vi "Properties_Update RW From Value.vi"(11 "Properties for Tree In":T1(array[cluster])=[{"Label"="a", "Tag"="a", "Property Type"=enum."Base", "Indent"=0, "Can Read?"=TRUE, "Can Write?"=TRUE, "Is Read?"=FALSE, "Is Write?"=TRUE, "Inactive Parent?"=FALSE, "Unwired?"=FALSE}, {"Label"="b", "Tag"="b", "Property Type"=enum."Scripting", "Indent"=0, "Can Read?"=TRUE, "Can Write?"=FALSE, "Is Read?"=FALSE, "Is Write?"=FALSE, "Inactive Parent?"=FALSE, "Unwired?"=FALSE}, {"Label"="c", "Tag"="c", "Property Type"=enum."Base", "Indent"=0, "Can Read?"=TRUE, "Can Write?"=TRUE, "Is Read?"=FALSE, "Is Write?"=FALSE, "Inactive Parent?"=FALSE, "Unwired?"=FALSE}, {"Label"="d", "Tag"="d", "Property Type"=enum."Private", "Indent"=0, "Can Read?"=TRUE, "Can Write?"=FALSE, "Is Read?"=FALSE, "Is Write?"=FALSE, "Inactive Parent?"=FALSE, "Unwired?"=FALSE}, {"Label"="E", "Tag"="E", "Property Type"=enum."Base", "Indent"=0, "Can Read?"=TRUE, "Can Write?"=TRUE, "Is Read?"=FALSE, "Is Write?"=TRUE, "Inactive Parent?"=FALSE, "Unwired?"=FALSE}, {"Label"="f", "Tag"="f", "Property Type"=enum."Base", "Indent"=0, "Can Read?"=TRUE, "Can Write?"=FALSE, "Is Read?"=FALSE, "Is Write?"=FALSE, "Inactive Parent?"=FALSE, "Unwired?"=FALSE}]) -> (3 "Properties for Tree Out":T1(array[cluster])=[{"Label"="a", "Tag"="a", "Property Type"=enum."Base", "Indent"=0, "Can Read?"=TRUE, "Can Write?"=TRUE, "Is Read?"=FALSE, "Is Write?"=TRUE, "Inactive Parent?"=FALSE, "Unwired?"=FALSE}, {"Label"="b", "Tag"="b", "Property Type"=enum."Scripting", "Indent"=0, "Can Read?"=TRUE, "Can Write?"=FALSE, "Is Read?"=FALSE, "Is Write?"=FALSE, "Inactive Parent?"=FALSE, "Unwired?"=FALSE}, {"Label"="c", "Tag"="c", "Property Type"=enum."Base", "Indent"=0, "Can Read?"=TRUE, "Can Write?"=TRUE, "Is Read?"=FALSE, "Is Write?"=FALSE, "Inactive Parent?"=FALSE, "Unwired?"=FALSE}, {"Label"="d", "Tag"="d", "Property Type"=enum."Private", "Indent"=0, "Can Read?"=TRUE, "Can Write?"=FALSE, "Is Read?"=FALSE, "Is Write?"=FALSE, "Inactive Parent?"=FALSE, "Unwired?"=FALSE}, {"Label"="E", "Tag"="E", "Property Type"=enum."Base", "Indent"=0, "Can Read?"=TRUE, "Can Write?"=TRUE, "Is Read?"=FALSE, "Is Write?"=TRUE, "Inactive Parent?"=FALSE, "Unwired?"=FALSE}, {"Label"="f", "Tag"="f", "Property Type"=enum."Base", "Indent"=0, "Can Read?"=TRUE, "Can Write?"=FALSE, "Is Read?"=FALSE, "Is Write?"=FALSE, "Inactive Parent?"=FALSE, "Unwired?"=FALSE}])   [LabVIEW 2023]
doc: "Update properties array with current R/W status based on selection values.\n\nIf trees aren't already populated, the properties array is passed thorugh without change."
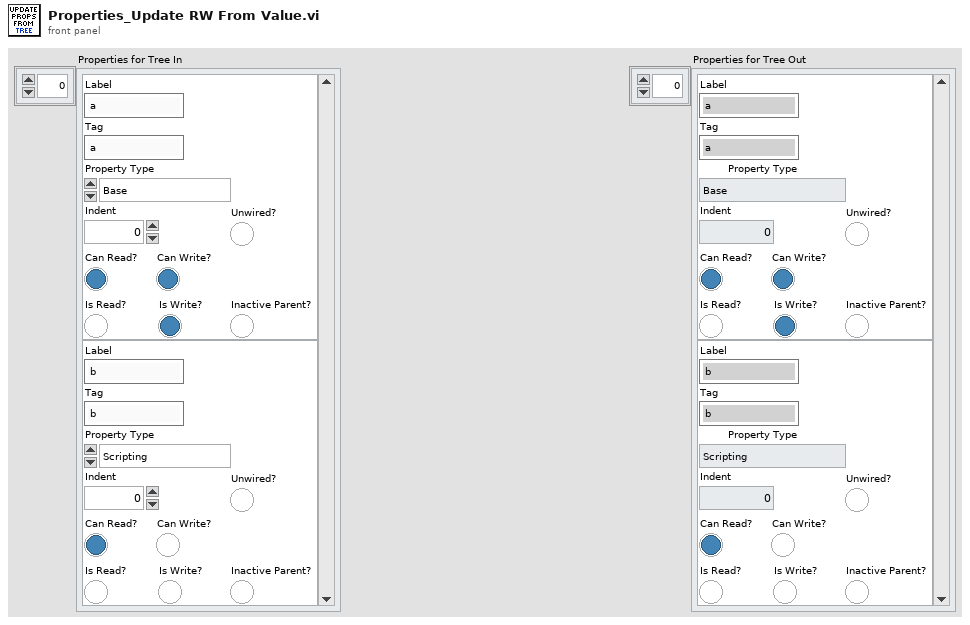
[diagram p1: front panel]
types:
  T1 = cluster{"Label":string, "Tag":string, "Property Type":enum16{"Unknown", "Base", "Scripting", "Private", "Deprecated", "None", "Divider"}, "Indent":u16, "Can Read?":bool, "Can Write?":bool, "Is Read?":bool, "Is Write?":bool, "Inactive Parent?":bool, "Unwired?":bool}[]
  T2 = enum16{"Init", "Read", "Remove", "Remove or Append", "Append", "Append If New"}
  T3 = cluster{"Tag":string, "Read":bool, "Write":bool, "New":bool}[]
  T4 = cluster{"Label":string, "Tag":string, "Property Type":enum16{"Unknown", "Base", "Scripting", "Private", "Deprecated", "None", "Divider"}, "Indent":u16, "Can Read?":bool, "Can Write?":bool, "Is Read?":bool, "Is Write?":bool, "Inactive Parent?":bool, "Unwired?":bool}
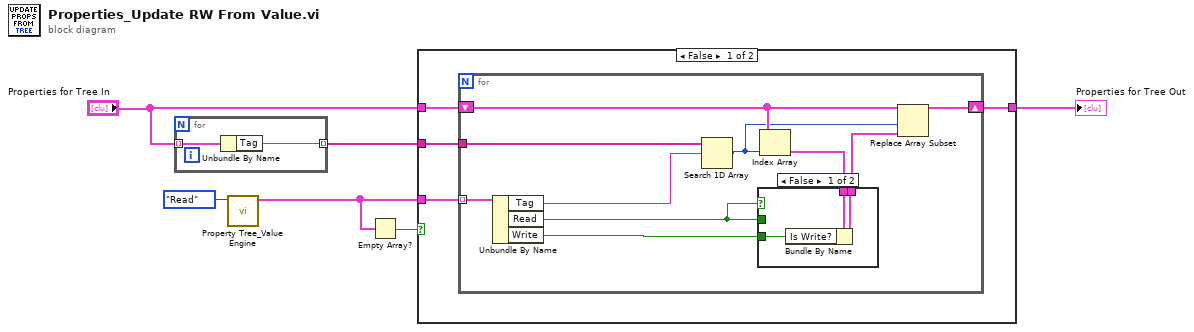
[diagram p0: block diagram]
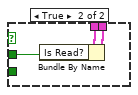
[diagram p2: hidden frame]
diagram:
  n1 = for {
    tunnel: "Properties for Tree In" -> [w8] mode=indexing
    tunnel: [w7] -> w3 mode=indexing
    n2 = Unbundle By Name(w8) -> ("Tag"=w7:string)
  }
  n3 = call "Property Tree_Value Engine.vi"("Save Action"=T2."Read" ("Action")) -> ("Property Array Out"=w1:T3)  [unwired: 8 in, 2 out]
  n4 = Empty Array?(array=w1) -> (empty?=w4:bool)
  n5 = case shown="False" w4 {
    tunnel: "Properties for Tree In" -> [w12 w29]
    tunnel: [w10 w29] -> w6
    tunnel: w3 -> [w11 _]
    tunnel: w1 -> [w9 _]
    frame False {
      n6 = for {
        tunnel: w11 -> [w22]
        shift-right: [w17] -> w10
        shift-left: w12 -> [w20]
        tunnel: w9 -> [w16] mode=indexing
        n7 = Unbundle By Name(w16) -> ("Tag"=w15:string, "Read"=w13:bool, "Write"=w14:bool)
        n8 = Search 1D Array(1D array=w22, element=w15) -> (index of element=w19:i32)  [unwired: 1 in]
        n9 = Index Array(array=w20, index=w19) -> (element=w21:T4)
        n10 = case shown="False" w13 {
          tunnel: w21 -> [w24 w28]
          tunnel: [w23 w27] -> w18
          tunnel: w13 -> [_ w26]
          tunnel: w14 -> [w25 _]
          frame False {
            n11 = Bundle By Name(cluster=w24, "Is Write?"=w25) -> (w23:T4)
          }
          frame True {
            n12 = Bundle By Name(cluster=w28, "Is Read?"=w26) -> (w27:T4)
          }
        }
        n13 = Replace Array Subset(array=w20, new element=w18, index=w19) -> (w17:T1)
      }
    }
    frame True {
    }
  }
  "Properties for Tree Out" <- w6
